vi "AB Tutorial GUI.vi"() -> ()   [LabVIEW 2019]
doc: "This VI provides an example application that can be used with the Application Builder documentation. Although the VI will run in Base, Full, and Professional versions of LabVIEW, the instructions in the LabVIEW Help are only usable when the Application Builder or Professional Development System are installed. Please refer to the LabVIEW Help topic on Application Builder for more information on how to use this example."
uses:
  <vilib>/Platform/browser.llb/Open URL in Default Browser (string).vi
panel:
  in  "Acquire Data":bool
  in  "Launch Tutorial":bool caption="Acquire Data"
  in  "prompt":string="Select location for datafile.txt..."
  out "Mode":dbl caption="Mode Value"
  out "Median":dbl caption="Median Value"
  out "Histogram":T1(graph)
  out "Mean":dbl caption="Mean Value"
  out "Standard \nDeviation":dbl
  in  "Type of Analysis":T2(radio)
  in  "Analyze Data":bool
  out "Points \nAcquired":i32
  out "Minimum":dbl
  out "Maximum":dbl
  in  "Graph Data":bool caption="Analyze  Data"
  in  "Quit":bool
  out "Data Display":dbl[][](graph)=[[-2.345731174920569, -0.0, 8.0], [0.3283775802120065, -4.135105280547405, 8.0], [-1.058242919077573, -7.5300212350454725, 8.0], [3.4294696501380444, -9.57705340788377, 8.0], [0.5142481273313284, -9.909780326907208, 8.0], [-0.23542019691068794, -8.468643432601228, 8.0], [8.146994228044576, -5.511608139186183, 8.0], [9.509734982087078, -1.567987683554373, 8.0], [2.445967845630477, 2.6563046457062844, 8.0], [-3.666544306815997, 6.405114922614751, 8.0], [-3.466658764889711, 9.007401138783667, 8.0], [-0.12754641902608815, 9.997350612346183, 8.0], [5.4241931074525365, 9.197761075416606, 8.0], [0.37878193978633323, 6.751760114912778, 8.0], [8.269555389908552, 3.0971851447908656, 8.0], [5.970714380774693, -1.1117900713797497, 8.0], [5.421376024291791, -5.121753391163054, 8.0], [6.673973498460271, -8.214916065354565, 8.0], [-0.8833352920224834, -9.837597875474406, 8.0], [-3.8948936024520804, -9.699336626744767, 8.0], [-5.721719841140654, -7.824881265945147, 8.0], [0.26078302104593193, -4.549761787135633, 8.0], [-5.399734292508953, -0.4602289179954143, 8.0], [2.3513343462771203, 3.7116855374714963, 8.0], [-2.8107495034960848, 7.2192033621168585, 8.0], [1.8781378229760204, 9.434474216326933, 8.0], [0.6534190430937608, 9.960961680990886, 8.0], [-1.4578140495013507, 8.704423802106659, 8.0], [-0.24090951183975132, 5.889782525459317, 8.0], [0.2527506657728119, 2.020862370205084, 8.0], [0.5772422965491537, -2.2097948278463977, 8.0], [-1.9245933421448105, -6.044895822764303, 8.0], [-3.580403264756872, -8.797952453264479, 8.0], [-0.26960141338017957, -9.976163933477718, 8.0], [-3.450829231271306, -9.368628846797973, 8.0], [-1.1342580884859408, -7.084096778991846, 8.0], [2.814639225689517, -3.5315019982053713, 8.0], [3.566211371957499, 0.6532363210516461, 8.0], [-1.8398866891603796, 4.721044473015279, 8.0], [3.438967582983176, 7.943779406850951, 8.0], [-2.727430245375383, 9.744567297862318, 8.0], [4.093692912544301, 9.80106472672314, 8.0], [5.261709920317863, 8.103158578783438, 8.0], [0.9781075274967616, 4.954776304996074, 8.0], [-6.879318326947709, 0.9194825053587801, 8.0], [1.8850650670342264, -3.2803998814560194, 8.0], [6.366452560974953, -6.89308634151903, 8.0], [-2.063621266203423, -9.271901210082097, 8.0], [2.722360155985981, -9.991033472697545, 8.0], [0.16678832967347015, -8.921757501190976, 8.0], [2.923970806799269, -6.255475111722558, -8.0], [1.796530594453417, -2.4694543860027935, -8.0], [-1.8473413816651356, 1.7586019479235433, -8.0], [1.0807119990695435, 5.671866202251332, -8.0], [0.8359518305868808, 8.569858888661317, -8.0], [2.1344061932507676, 9.933835475172536, -8.0], [5.616421823487202, 9.519642344931208, -8.0], [1.2904450192644363, 7.401420617238417, -8.0], [4.031445442013301, 3.958334788925615, -8.0], [-0.1264465180958026, -0.19329821313762774, -8.0], [-0.14406418915757044, -4.310330578844173, -8.0], [0.7352063544906724, -7.655808057855752, -8.0], [-6.181662430891462, -9.63088574720172, -8.0], [-0.14754766762488258, -9.882022122643413, -8.0], [-0.5145052458603931, -8.364263440110719, -8.0], [0.10945026215546814, -5.349290515474121, -8.0], [1.860117068641511, -1.3767874984073882, -8.0], [-3.9596790205091135, 2.8421623057226593, -8.0], [-7.693199854431916, 6.552361290014491, -8.0], [-0.7716861422137945, 9.089678918636091, -8.0], [5.801723924216416, 9.999931973003505, -8.0], [3.28298592915856, 9.120183949899731, -8.0], [0.7420201437043115, 6.607910911512985, -8.0], [-0.5715064116858415, 2.9128130615801333, -8.0], [-9.334147557818541, -1.303682187132679, -8.0], [1.1930589394631002, -5.286816596397042, -8.0], [0.7301852760646194, -8.32360382755146, -8.0], [4.298089537062088, -9.870454941141936, -8.0], [-3.514834932667216, -9.65048153757839, -8.0], [-0.17472032245797317, -7.703059147660099, -8.0], [0.07059573070625538, -4.376778960372741, -8.0], [1.4224564432577216, -0.2670495380235618, -8.0], [0.6534140854313512, 3.890482105589872, -8.0], [7.260366070643439, 7.351612295704545, -8.0], [-1.162790780651353, 9.496794140771671, -8.0], [0.34012487934849345, 9.942037247215818, -8.0], [3.192617750430069, 8.60764250884073, -8.0], [1.740446818945077, 5.732468352474828, -8.0], [3.2172166043054258, 1.8311747629766575, -8.0], [4.54578568800855, -2.3979015362053997, -8.0], [-0.24218677459074442, -6.197750282133645, -8.0], [0.6463081736654654, -8.88819351281767, -8.0], [1.718081190051713, -9.987638323945728, -8.0], [8.790710701755284, -9.299282637078395, -8.0], [-1.4834769902017186, -6.946343032538707, -8.0], [-3.4753056770536412, -3.349998818217993, -8.0], [5.2680448645685845, 0.845999624784014, -8.0], [-6.106626553434015, 4.890563013628535, -8.0], [3.538568606473051, 8.05970914088876, -8.0], [-1.27718053229108, 9.786156649274032, -8.0], [-4.050800631432669, 9.760869146481934, 8.0], [3.5657991326739613, 7.988373129029302, 8.0], [-6.722259698248682, 4.785947733376119, 8.0], [-3.640732427316833, 0.7268313499650346, 8.0], [-1.9014346234410495, -3.462388808460615, 8.0], [0.5286482652424748, -7.031836780985426, 8.0], [-0.22453299909719956, -9.342576649440492, 8.0], [-2.40614209621282, -9.980982914626752, 8.0], [-3.3159196448032726, -8.832780008907084, 8.0], [-2.761637397811836, -6.1034977742786864, 8.0], [0.164849553697862, -2.2816813482380898, 8.0], [-1.5138163802730902, 1.9485590633674268, 8.0], [-2.436639775598557, 5.830004819933208, 8.0], [0.035682361792854375, 8.667871986413065, 8.0], [-5.111401373514437, 9.954178578586143, 8.0], [4.821883667689623, 9.458674011532096, 8.0], [0.4586429207206388, 7.2700542595148265, 8.0], [-6.149510677697306, 3.78008515902829, 8.0], [0.12451236775319048, -0.38652419519807313, 8.0], [3.439580574498151, -4.483945206169529, 8.0], [3.4885488214290166, -7.7787340820391755, 8.0], [5.082976990295504, -9.681119246983364, 8.0], [4.449290163760889, -9.850571234980892, 8.0], [2.31131602484374, -8.256757915581868, 8.0], [0.489202733369629, -5.184973985461696, 8.0], [-0.46527048712733454, -1.185072839575157, 8.0], [1.2237500975472622, 3.02695791533754, 8.0], [-5.969672949416895, 6.697159191355555, 8.0], [2.035540531204822, 9.168560095442496, 8.0], [-2.163201720790416, 9.99877659007466, 8.0], [0.22239466433186558, 9.03919882231129, 8.0], [-5.633256092073918, 6.461592484444154, 8.0], [0.022997941566310583, 2.727352527412474, 8.0], [1.181789337238264, -1.495087146966525, 8.0], [-1.1433660533876349, -5.449904240391142, 8.0], [-3.7405217239365536, -8.42918125126803, 8.0], [-1.4664693536432927, -9.899623645799267, 8.0], [0.9767673181638841, -9.59802028638147, 8.0], [0.09308858005297344, -7.578358574107382, 8.0], [-0.8938341469279198, -4.202160632413216, 8.0], [0.10673419627864124, -0.07377036780799094, 8.0], [0.6580069148765367, 4.06782489041308, 8.0], [3.354633653755929, 7.481274101594879, 8.0], [0.8567418462985185, 9.555565332615984, 8.0], [2.3577350415381075, 9.91939770377628, 8.0], [-0.2942859624038727, 8.507644738400359, 8.0], [-2.8261229106978734, 5.573012088483433, 8.0], [1.704357948191508, 1.6408028880383807, 8.0], [5.805607080213574, -2.585112204150357, 8.0], [0.05417482294967114, -6.348288785386675, 8.0], [-3.6978171333783383, -8.975113259766822, -8.0], [-0.8739640559372153, -9.995380564680246, -8.0], [0.4856101937579671, -9.22646150024496, -8.0], [-4.953966149214734, -6.805993598150404, -8.0], [2.4781112109594967, -3.167243821055114, -8.0], [3.663336126244416, 1.038446797998695, -8.0], [6.789285334318091, 5.058254063812468, -8.0], [3.8113384043894545, 8.172627147794813, -8.0], [1.1925390114817802, 9.824089139999986, -8.0], [-1.5017211699505655, 9.717026154910645, -8.0], [-0.4605334158384764, 7.870602608763184, -8.0], [0.7305071619374819, 4.615330763640587, -8.0], [1.991878092975903, 0.5339085944852254, -8.0], [0.015338830358053251, -3.643083920746595, -8.0], [-2.3207262087616987, -7.167959585477776, -8.0], [5.549700732701033, -9.409760983712602, -8.0], [0.46098095664132077, -9.967202693795189, -8.0], [1.8774830018424793, -8.740501910765532, -8.0], [-3.7339948990952414, -5.949239700703501, -8.0], [-2.607534024534238, -2.0930556988590237, -8.0], [3.399989474805755, 2.1377880472997846, -8.0], [-2.391206420293749, 5.98596489948335, -8.0], [1.3267493243101027, 8.762646100625851, -8.0], [-2.395233927758824, 9.970802035400212, -8.0], [-0.2909734822248203, 9.394171190144299, -8.0], [-2.092620564320428, 7.135971250448213, -8.0], [-1.46263588222889, 3.600422998624527, -8.0], [3.1280741284873135, -0.579605742095239, -8.0], [4.189468923297554, -4.655884286747688, -8.0], [-7.39303218200613, -7.898753372979966, -8.0], [0.9274789771052246, -9.72773513613017, -8.0], [-0.39222379369570226, -9.815439416389857, -8.0], [-1.040457589437915, -8.146167031345925, -8.0], [-7.982853863684959, -5.018719950440453, -8.0], [-0.09142453465739832, -0.9929153463972145, -8.0], [0.16314570481060012, 3.210622420700217, -8.0], [-5.9215673649098175, 6.839454519007056, -8.0], [-1.6077373860561481, 9.24401519312921, -8.0], [1.455956161563944, 9.99388489529956, -8.0], [-7.5425380260740145, 8.95483595492273, -8.0], [-4.753832521677461, 6.312859509522612, -8.0], [-3.2146810739736, 2.540872844605415, -8.0], [-1.6923016300331717, -1.6859334272690527, -8.0], [0.5936702177597443, -5.610955381059939, -8.0], [-4.0278169343724715, -8.531608884659791, -8.0], [0.5890894552877117, -9.925093089775237, -8.0], [-4.446709771403941, -9.541972476711742, -8.0], [-6.925737445154908, -7.4508261430108425, -8.0], [-3.9434566886622107, -4.025972054092693, -8.0], [-1.9437150094830526, 0.11953636869005169, -8.0]]
  # "Instructions"
  # "This VI is part of the Application Builder Tutorial.  If you would like to learn more about the LabVIEW Application Builder by using this tutorial, click \"Launch Tutorial\" below."
  # "Step 1"
  # "Generate data to be analyzed.  Each push of the button will create additional data."
  # "Step 2"
  # "Show the acquired data, a sine wave, and data read from a file."
  # "Step 3"
  # "Analyze the data.  Select the type of analysis you want to perform and click \"Analyze\"."
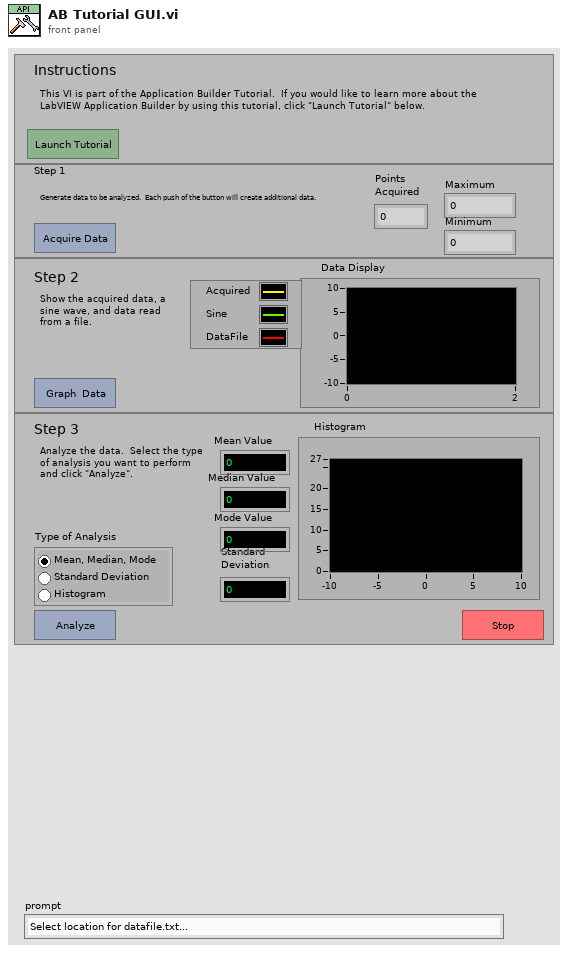
[diagram p1: front panel]
types:
  T1 = cluster{"X Values":dbl[], "Histogram: h(x)":i32[]}
  T2 = enum32{"Mean-Med-Mode", "Standard Deviation", "Histogram"}
  T3 = enum32{"invalid app kind", "Development System", "Run Time System", "Student Edition", "Embedded LabVIEW", "Evaluation", "Custom"}
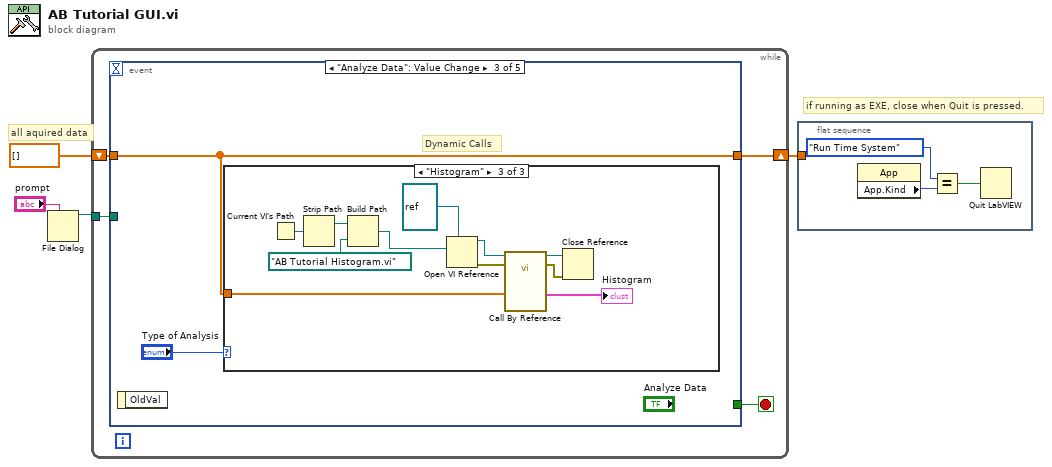
[diagram p0: block diagram]
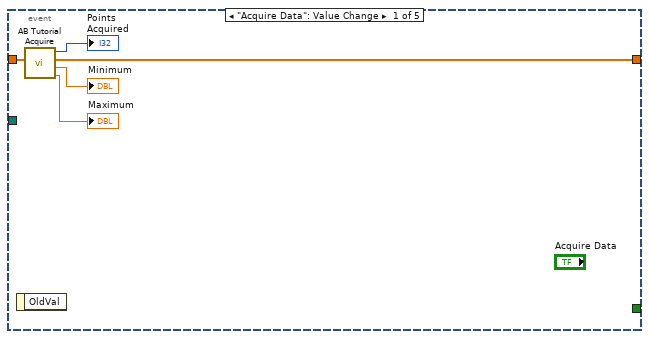
[diagram p2: hidden frame]
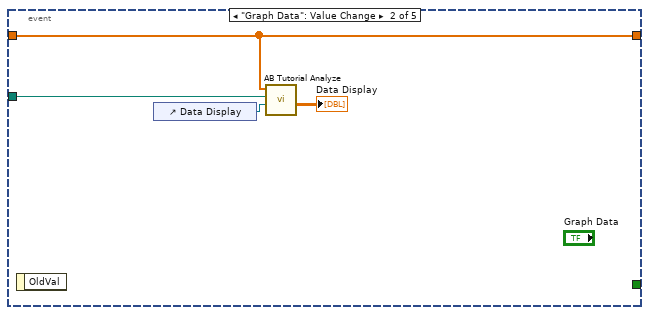
[diagram p3: hidden frame]
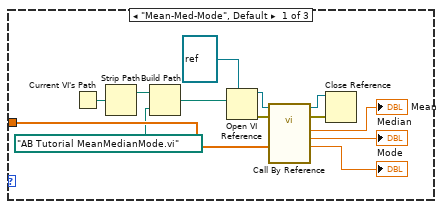
[diagram p4: hidden frame]
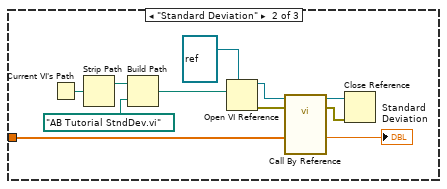
[diagram p5: hidden frame]
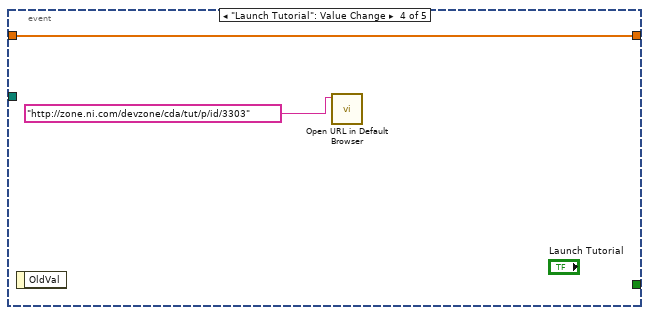
[diagram p6: hidden frame]
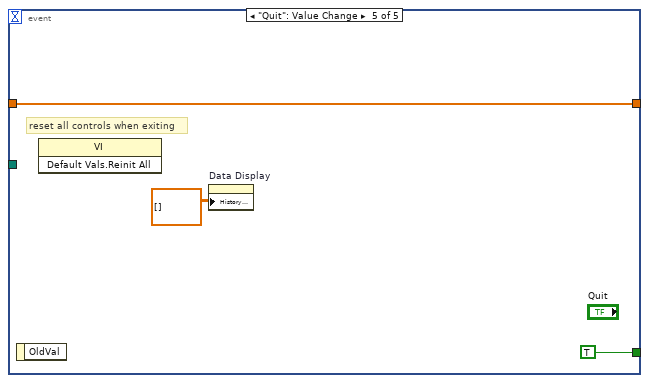
[diagram p7: hidden frame]
diagram:
  # "if running as EXE, close when Quit is pressed."
  # "all aquired data"
  n1 = File Dialog(7:"prompt") -> (3:w3:path)  [unwired: 6 in, 3 out]
  n2 = while {
    shift-right: [w6] -> w1
    shift-left: dbl[] [] ("Array Out") -> [w7]
    tunnel: w3 -> [w5]
    stop <- w8 stop-if-true
    n3 = event shown="[2] \"Analyze Data\": Value Change" {
      selector: _ -> [_ _ _ _ _]
      dyn-events: _ -> [_ _ _ _ _]
      timeout: _ -> [_ _ _ _ _]
      tunnel: [_ _ _ _ TRUE ("Value")] -> w8
      tunnel: w7 -> [w13 w16 w19 w56 w59]
      tunnel: [w11 w16 w19 w56 w59] -> w6
      tunnel: w5 -> [_ w17 _ _ _]
      event "Acquire Data": Value Change {
        n4 = event-data() -> ()  [unwired: 1 in, 1 out]
        n5 = call "AB Tutorial Acquire.vi"("Array In"=w13) -> ("Max"=→"Maximum":dbl, "Min"=→"Minimum":dbl, "Array Out"=w11:dbl[], "# points acquired"=→"Points \nAcquired":i32)  [unwired: 7 in]
      }
      event "Graph Data": Value Change {
        n6 = event-data() -> ()  [unwired: 1 in, 1 out]
        n7 = control-ref of="Data Display"() -> (w15:refnum<vi>)
        n8 = call "AB Tutorial Analyze.vi"("WFChart Refnum"=w15, "Datafile path"=w17, "Array In"=w16) -> ("Array Out"=→"Data Display":dbl[][])  [unwired: 8 in]
      }
      event "Analyze Data": Value Change {
        # "Dynamic Calls"
        n9 = event-data() -> ()  [unwired: 1 in, 1 out]
        n10 = case shown="\"Histogram\"" "Type of Analysis" {
          tunnel: w19 -> [w29 w37 w48]
          frame "Mean-Med-Mode", Default {
            n11 = Current VI's Path() -> (path=w28:path)
            n12 = Strip Path(path=w28) -> (stripped path=w27:path)  [unwired: 1 out]
            n13 = Build Path(base path=w27, name or relative path=path "AB Tutorial MeanMedianMode.vi") -> (appended path=w26:path)
            n14 = Open VI Reference(type specifier VI Refnum (for type only)=refnum<vi> refnum, vi path=w26) -> (vi reference=w31:refnum<vi>, error out=w32:errorcluster)  [unwired: 4 in]
            n15 = call-by-ref "?"(reference=w31, error in=w32, "Array"=w29) -> (reference out=w24:refnum<vi>, error out=w25:errorcluster, "mode"=→"Mode":dbl, "median"=→"Median":dbl, "mean"=→"Mean":dbl)  [unwired: 8 in]
            n16 = Close Reference(reference=w24, error in (no error)=w25) -> ()  [unwired: 1 out]
          }
          frame "Standard Deviation" {
            n17 = Current VI's Path() -> (path=w40:path)
            n18 = Strip Path(path=w40) -> (stripped path=w39:path)  [unwired: 1 out]
            n19 = Build Path(base path=w39, name or relative path=path "AB Tutorial StndDev.vi") -> (appended path=w38:path)
            n20 = Open VI Reference(type specifier VI Refnum (for type only)=refnum<vi> refnum, vi path=w38) -> (vi reference=w42:refnum<vi>, error out=w43:errorcluster)  [unwired: 4 in]
            n21 = call-by-ref "?"(reference=w42, error in=w43, "Array"=w37) -> (reference out=w36:refnum<vi>, error out=w33:errorcluster, "standard deviation"=→"Standard \nDeviation":dbl)  [unwired: 10 in]
            n22 = Close Reference(reference=w36, error in (no error)=w33) -> ()  [unwired: 1 out]
          }
          frame "Histogram" {
            n23 = Current VI's Path() -> (path=w51:path)
            n24 = Strip Path(path=w51) -> (stripped path=w50:path)  [unwired: 1 out]
            n25 = Build Path(base path=w50, name or relative path=path "AB Tutorial Histogram.vi") -> (appended path=w49:path)
            n26 = Open VI Reference(type specifier VI Refnum (for type only)=refnum<vi> refnum, vi path=w49) -> (vi reference=w53:refnum<vi>, error out=w54:errorcluster)  [unwired: 4 in]
            n27 = call-by-ref "?"(reference=w53, error in=w54, "Array"=w48) -> (reference out=w47:refnum<vi>, error out=w46:errorcluster, "Cluster"=→"Histogram":T1)  [unwired: 10 in]
            n28 = Close Reference(reference=w47, error in (no error)=w46) -> ()  [unwired: 1 out]
          }
        }
      }
      event "Launch Tutorial": Value Change {
        n29 = event-data() -> ()  [unwired: 1 in, 1 out]
        n30 = call-poly <vilib>:"Open URL in Default Browser.vi"("URL"="http://zone.ni.com/devzone/cda/tut/p/id/3303" ("HTML filename")) -> ()  [unwired: 5 in, 2 out]
      }
      event "Quit": Value Change {
        # "reset all controls when exiting"
        n31 = event-data() -> ()  [unwired: 1 in, 1 out]
        n32 = invoke class="VI" method="Default Vals.Reinit All"() -> ()  [unwired: 3 in, 3 out]
        n33 = property on="Data Display" class="WFChart (strict)"("History Data"=dbl[][] []) -> ()  [unwired: 2 in, 2 out]
      }
    }
  }
  n34 = flat-sequence {
    tunnel: w1 -> [_]
    frame #0 {
      n35 = property class="App"() -> ("App.Kind"=w62:T3)  [unwired: 2 in, 2 out]
      n36 = Equal?(x=T3."Run Time System" ("Application:Kind"), y=w62) -> (x = y?=w60:bool)
      n37 = Quit LabVIEW(quit? (T)=w60) -> ()
    }
  }
